vi "Test Config Enabler.vi"(0 "StringRefArray":refnum<vi>[](array[refnum]), 2 "Mode":enum16{"Init", "Enable", "Disable", "AutoPop"}(ring)=enum."Enable", 7 "TabRef":refnum<vi>, 9 "RadioButtonRef":refnum<vi>, 11 "TableRef":refnum<vi>) -> ()   [LabVIEW 2019]
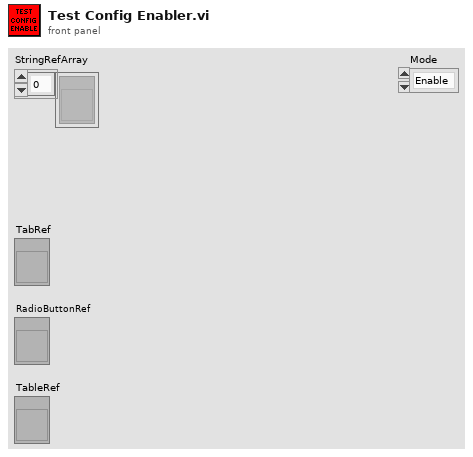
[diagram p1: front panel]
types:
  T1 = enum8{"Enabled", "Disabled", "Disabled and Grayed Out"}
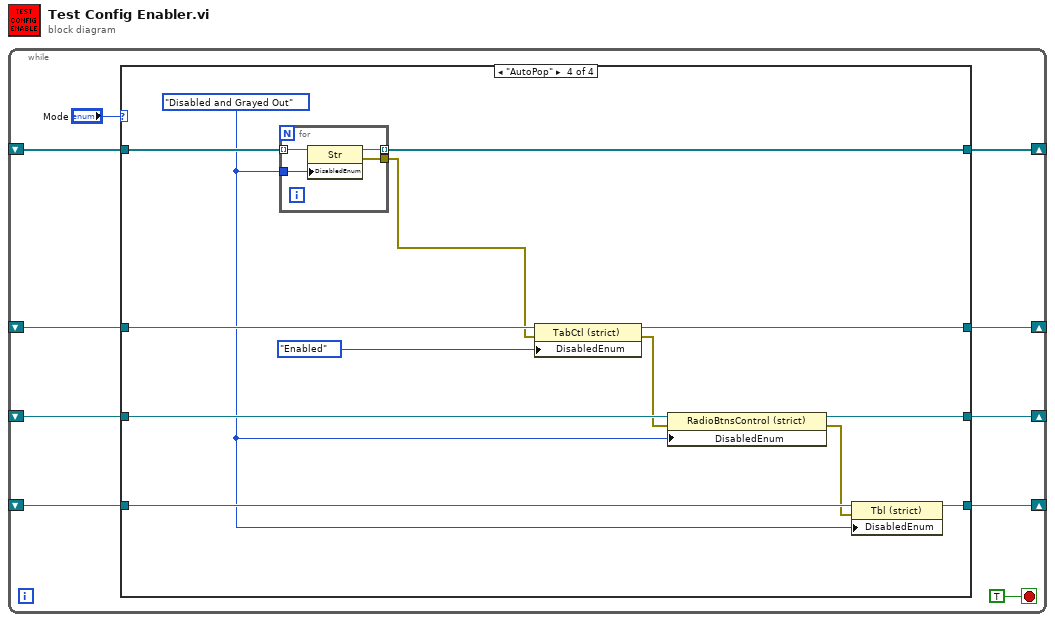
[diagram p0: block diagram]
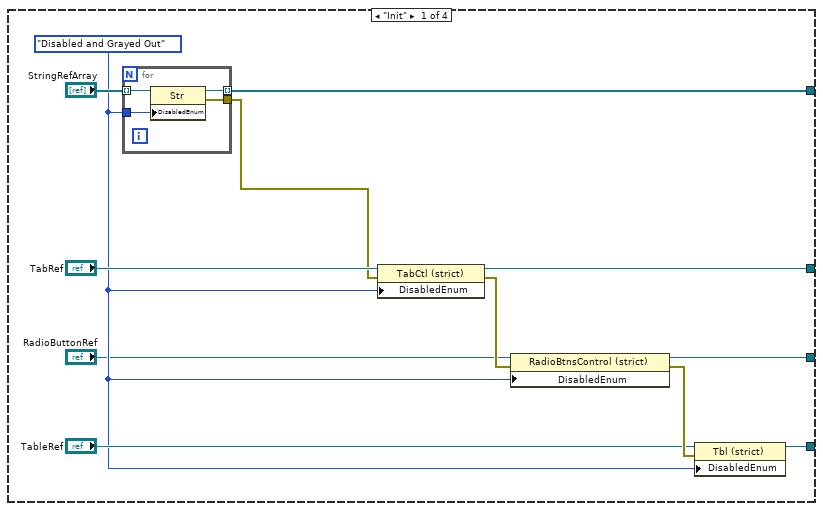
[diagram p2: hidden frame]
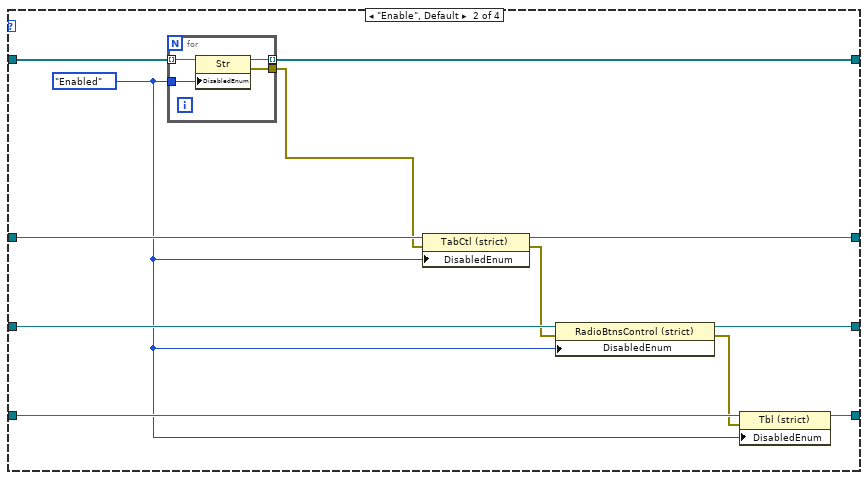
[diagram p3: hidden frame]
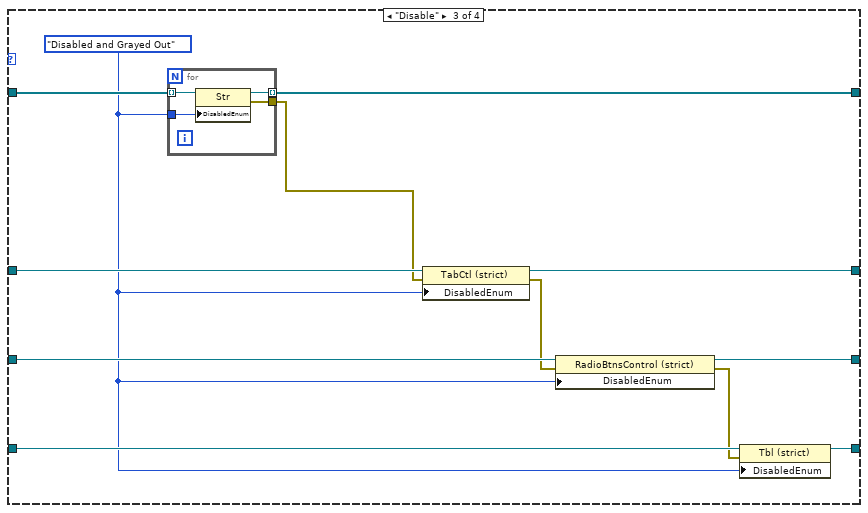
[diagram p4: hidden frame]
diagram:
  n1 = while {
    shift-right: [w8] -> _
    shift-left: _ -> [w4]
    shift-right: [w7] -> _
    shift-left: _ -> [w3]
    shift-right: [w6] -> _
    shift-left: _ -> [w2]
    shift-right: [w5] -> _
    shift-left: _ -> [w1]
    stop <- TRUE stop-if-true
    n2 = case shown="\"AutoPop\"" "Mode" {
      tunnel: [w14 w31 w47 w64] -> w8
      tunnel: [w16 w32 w48 w65] -> w7
      tunnel: [w18 w33 w49 w66] -> w6
      tunnel: [w20 w34 w50 w67] -> w5
      tunnel: w4 -> [_ w38 w54 w71]
      tunnel: w3 -> [_ w37 w53 w70]
      tunnel: w2 -> [_ w36 w52 w69]
      tunnel: w1 -> [_ w35 w51 w68]
      frame "Init" {
        w13 = T1."Disabled and Grayed Out" ("Enabled State")
        n3 = for {
          tunnel: "StringRefArray" -> [w26] mode=indexing
          tunnel: [w25] -> w12
          tunnel: [w24] -> w14 mode=indexing
          tunnel: w13 -> [w23]
          n4 = property on="Property Node" class="Str"(reference=w26, "DisabledEnum"=w23) -> (reference out=w24:refnum<vi>, error out=w25:errorcluster)  [unwired: 1 in]
        }
        n5 = property on="Property Node" class="TabCtl (strict)"(reference="TabRef", error in=w12, "DisabledEnum"=w13) -> (reference out=w16:refnum<vi>, error out=w22:errorcluster)
        n6 = property on="Property Node" class="RadioBtnsControl (strict)"(reference="RadioButtonRef", error in=w22, "DisabledEnum"=w13) -> (reference out=w18:refnum<vi>, error out=w21:errorcluster)
        n7 = property on="Property Node" class="Tbl (strict)"(reference="TableRef", error in=w21, "DisabledEnum"=w13) -> (reference out=w20:refnum<vi>)  [unwired: 1 out]
      }
      frame "Enable", Default {
        w27 = T1."Enabled" ("Enabled State")
        n8 = for {
          tunnel: w38 -> [w42] mode=indexing
          tunnel: [w41] -> w28
          tunnel: [w40] -> w31 mode=indexing
          tunnel: w27 -> [w39]
          n9 = property on="Property Node" class="Str"(reference=w42, "DisabledEnum"=w39) -> (reference out=w40:refnum<vi>, error out=w41:errorcluster)  [unwired: 1 in]
        }
        n10 = property on="Property Node" class="TabCtl (strict)"(reference=w37, error in=w28, "DisabledEnum"=w27) -> (reference out=w32:refnum<vi>, error out=w30:errorcluster)
        n11 = property on="Property Node" class="RadioBtnsControl (strict)"(reference=w36, error in=w30, "DisabledEnum"=w27) -> (reference out=w33:refnum<vi>, error out=w29:errorcluster)
        n12 = property on="Property Node" class="Tbl (strict)"(reference=w35, error in=w29, "DisabledEnum"=w27) -> (reference out=w34:refnum<vi>)  [unwired: 1 out]
      }
      frame "Disable" {
        w43 = T1."Disabled and Grayed Out" ("Enabled State")
        n13 = for {
          tunnel: w54 -> [w58] mode=indexing
          tunnel: [w57] -> w44
          tunnel: [w56] -> w47 mode=indexing
          tunnel: w43 -> [w55]
          n14 = property on="Property Node" class="Str"(reference=w58, "DisabledEnum"=w55) -> (reference out=w56:refnum<vi>, error out=w57:errorcluster)  [unwired: 1 in]
        }
        n15 = property on="Property Node" class="TabCtl (strict)"(reference=w53, error in=w44, "DisabledEnum"=w43) -> (reference out=w48:refnum<vi>, error out=w46:errorcluster)
        n16 = property on="Property Node" class="RadioBtnsControl (strict)"(reference=w52, error in=w46, "DisabledEnum"=w43) -> (reference out=w49:refnum<vi>, error out=w45:errorcluster)
        n17 = property on="Property Node" class="Tbl (strict)"(reference=w51, error in=w45, "DisabledEnum"=w43) -> (reference out=w50:refnum<vi>)  [unwired: 1 out]
      }
      frame "AutoPop" {
        w59 = T1."Disabled and Grayed Out" ("Enabled State")
        n18 = for {
          tunnel: w71 -> [w75] mode=indexing
          tunnel: [w74] -> w61
          tunnel: [w73] -> w64 mode=indexing
          tunnel: w59 -> [w72]
          n19 = property on="Property Node" class="Str"(reference=w75, "DisabledEnum"=w72) -> (reference out=w73:refnum<vi>, error out=w74:errorcluster)  [unwired: 1 in]
        }
        n20 = property on="Property Node" class="TabCtl (strict)"(reference=w70, error in=w61, "DisabledEnum"=T1."Enabled" ("Enabled State")) -> (reference out=w65:refnum<vi>, error out=w63:errorcluster)
        n21 = property on="Property Node" class="RadioBtnsControl (strict)"(reference=w69, error in=w63, "DisabledEnum"=w59) -> (reference out=w66:refnum<vi>, error out=w62:errorcluster)
        n22 = property on="Property Node" class="Tbl (strict)"(reference=w68, error in=w62, "DisabledEnum"=w59) -> (reference out=w67:refnum<vi>)  [unwired: 1 out]
      }
    }
  }
